vi "Calibration Axis.vi"() -> ()   [LabVIEW 2016]
doc: "This example builds a local coordinate system based on the information returned by an X-Y-Theta positioning system. The example finds the location of the template in the image and transforms the coordinates from the image coordinate system to the local system using the IMAQ Convert Pixel to Real World VI."
uses:
  <vilib>/vision/Calibration.llb/Error Statistics.ctl
  <vilib>/vision/NI_Vision_Development_Module.lvlib
panel:
  out "Calibration Axis Info":T1={"Origin Pixel"={"X"=0.0, "Y"=0.0}, "Angle Relative to Horizontal (deg)"=0.0, "X Axis Pixel"={"X"=0.0, "Y"=0.0}, "Axis Reference"=1} {"X Axis Pixel"."Y" format="%.2f"; "X Axis Pixel"."X" format="%.2f"; "Axis Reference" items=["Direct", "Indirect"]; "Angle Relative to Horizontal (deg)" format="%.2f"; "Origin Pixel"."Y" format="%.2f"; "Origin Pixel"."X" format="%.2f"}
  out "Error Statistics":T2
  out "Error Map":sgl[][](array[numeric]) format="%.2f"
  out "Board Mounting \nHole Location":T3 {"Calibration Axis (mm)"."Y" format="%#_2g"; "Calibration Axis (mm)"."X" format="%#_2g"}
  out "Calibration Axis":T4={"Origin Point (pixels)"={"X"=0.0, "Y"=0.0}, "Angle (degrees)"=0.0, "Axis Reference"=1} {"Axis Reference" items=["Direct", "Indirect"]; "Angle (degrees)" format="%.2f"; "Origin Point (pixels)"."Y" format="%.2f"; "Origin Point (pixels)"."X" format="%.2f"}
  out "Board Corner Template":T5(plugin-control)
  out "Mounting Hole Template":T5(plugin-control)
  out "Image":T5(plugin-control)
  # "Overview: Demonstrates how to use the Calibration functions to apply a simple calibration to an image, update the calibration axis as the part moves, and calculate the real world position of a feature compared with the pixel position of that same feature. \nRequirements: Vision Development Software.\nInstructions: Run the VI."
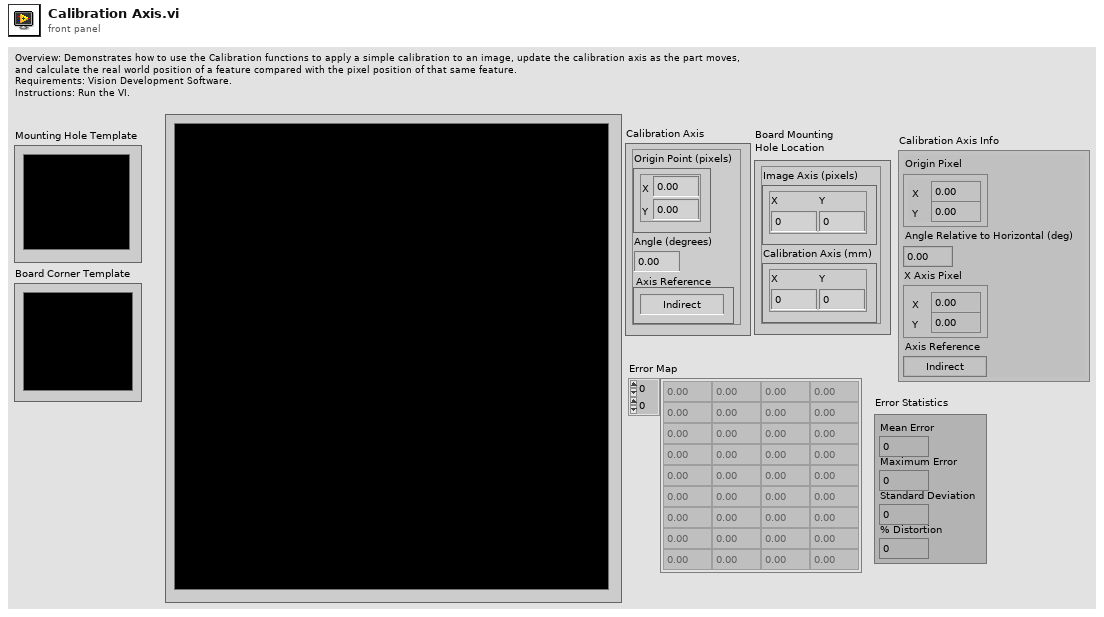
[diagram p1: front panel]
types:
  T1 = cluster{"Origin Pixel":cluster{"X":sgl, "Y":sgl}, "Angle Relative to Horizontal (deg)":sgl, "X Axis Pixel":cluster{"X":sgl, "Y":sgl}, "Axis Reference":u32}
  T2 = typedef "Error Statistics.ctl" = cluster{"Mean Error":dbl, "Maximum Error":dbl, "Standard Deviation":dbl, "% Distortion":dbl}
  T3 = cluster{"Image Axis (pixels)":cluster{"X":dbl, "Y":dbl}, "Calibration Axis (mm)":cluster{"X":dbl, "Y":dbl}}
  T4 = cluster{"Origin Point (pixels)":cluster{"X":sgl, "Y":sgl}, "Angle (degrees)":sgl, "Axis Reference":u32}
  T5 = typedef "IMAQ Image.ctl" = refnum<image>
  T6 = typedef "Image Type" = u32
  T7 = typedef "Simple Grid Descriptor" = cluster{"X Step":sgl, "Y Step":sgl, "Unit":T8}
  T8 = typedef "Image Unit" = enum32{"Undefined", "Angström", "Micrometer", "Millimeter", "Centimeter", "Meter", "Kilometer", "Microinch", "Inch", "Feet", "Nautical miles", "Standard miles", "Steps"}
  T9 = cluster{"Number of Matches Requested":i32, "Minimum Match Score":sgl, "Angle Ranges":cluster{"Start Angle":sgl, "End Angle":sgl}[]}
  T10 = cluster{"Position":cluster{"x":sgl, "y":sgl}, "Angle":sgl, "Scale":sgl, "Score":sgl, "Bounding Box":cluster{"x":sgl, "y":sgl}[]}[]
  T11 = cluster{"Position":cluster{"x":sgl, "y":sgl}, "Angle":sgl, "Scale":sgl, "Score":sgl, "Bounding Box":cluster{"x":sgl, "y":sgl}[]}
  T12 = cluster{"Position":cluster{"x":sgl, "y":sgl}, "Angle":sgl, "Axis Reference":u32}
  T13 = cluster{"Position":cluster{"x":sgl, "y":sgl}, "Real World Coordinates":cluster{"X":sgl, "Y":sgl}}
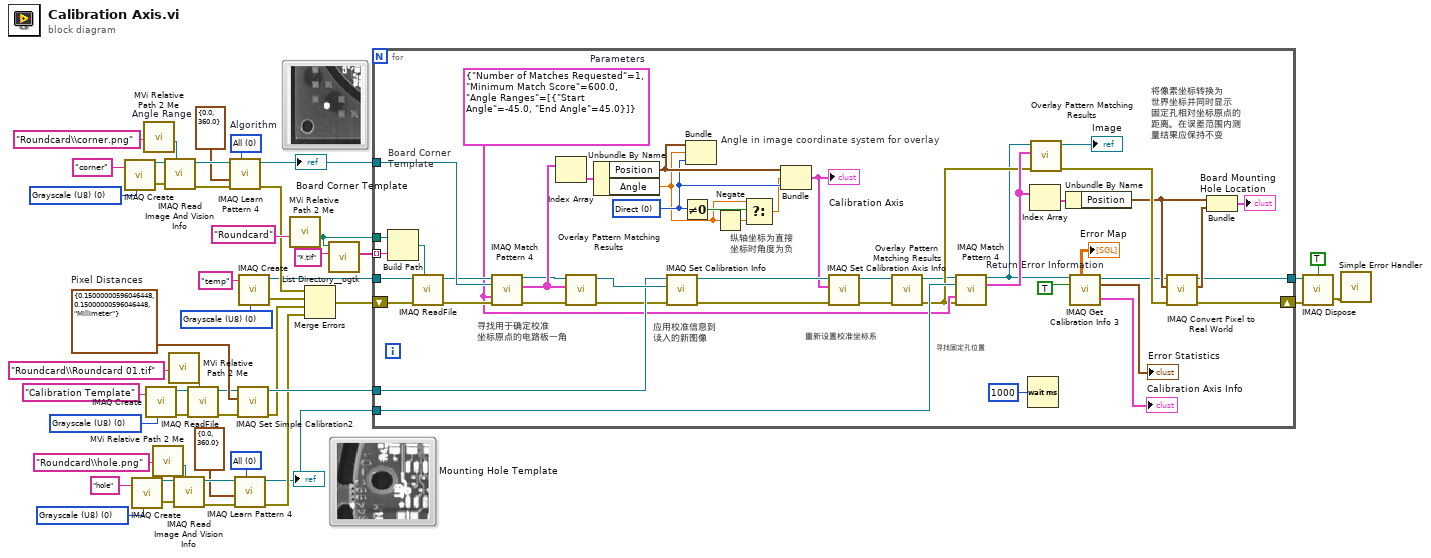
[diagram p0: block diagram]
diagram:
  w6 = 0 items=["All", "Low Discrepancy Sampling", "Grayscale Value Pyramid", "Gradients Pyramid"] ("Algorithm")
  w14 = T6 0 items=["Grayscale (U8)", "Grayscale (I16)", "Grayscale (SGL)", "Complex (CSG)", "RGB (U32)", "HSL (U32)", "RGB (U64)", "Grayscale (U16)"] ("Image Type")
  w24 = cluster{"Start Angle":sgl, "End Angle":sgl} {"Start Angle"=0.0, "End Angle"=360.0}  # Angle Range
  w7 = 0 items=["All", "Low Discrepancy Sampling", "Grayscale Value Pyramid", "Gradients Pyramid"]  # Algorithm
  w38 = T7 {"X Step"=0.15, "Y Step"=0.15, "Unit"=enum."Millimeter"}  # Pixel Distances
  w40 = T6 0 items=["Grayscale (U8)", "Grayscale (I16)", "Grayscale (SGL)", "Complex (CSG)", "RGB (U32)", "HSL (U32)", "RGB (U64)", "Grayscale (U16)"] ("Image Type")
  w43 = T6 0 items=["Grayscale (U8)", "Grayscale (I16)", "Grayscale (SGL)", "Complex (CSG)", "RGB (U32)", "HSL (U32)", "RGB (U64)", "Grayscale (U16)"] ("Image Type")
  w44 = T6 0 items=["Grayscale (U8)", "Grayscale (I16)", "Grayscale (SGL)", "Complex (CSG)", "RGB (U32)", "HSL (U32)", "RGB (U64)", "Grayscale (U16)"] ("Image Type")
  n1 = call "IMAQ Create"("Image Name"="corner" ("name or relative path"), "Image Type"=w43) -> ("Src"=w42:T5, "error out"=w41:errorcluster)  [unwired: 2 in, 1 out]
  n2 = call "IMAQ Create"("Image Name"="hole" ("name or relative path"), "Image Type"=w44) -> ("Src"=w47:T5, "error out"=w48:errorcluster)  [unwired: 2 in, 1 out]
  n3 = call "MVi Relative Path 2 Me.vi"("Relative Path"="Roundcard\\corner.png" ("name or relative path")) -> ("Appended Dir"=w20:path)  [unwired: 5 in, 1 out]
  n4 = call "IMAQ Create"("Image Name"="Calibration Template", "Image Type"=w40) -> ("Src"=w35:T5, "error out"=w32:errorcluster)  [unwired: 2 in, 1 out]
  n5 = call "MVi Relative Path 2 Me.vi"("Relative Path"="Roundcard\\hole.png" ("name or relative path")) -> ("Appended Dir"=w18:path)  [unwired: 5 in, 1 out]
  n6 = call "IMAQ Read Image And Vision Info"("File Path"=w20, "error in (no error)"=w41, "Image"=w42) -> ("error out"=w29:errorcluster, "Image Out"=w28:T5)  [unwired: 1 in, 6 out]
  n7 = call "MVi Relative Path 2 Me.vi"("Relative Path"="Roundcard\\Roundcard 01.tif" ("name or relative path")) -> ("Appended Dir"=w15:path)  [unwired: 5 in, 1 out]
  n8 = call "IMAQ Read Image And Vision Info"("File Path"=w18, "error in (no error)"=w48, "Image"=w47) -> ("error out"=w25:errorcluster, "Image Out"=w26:T5)  [unwired: 1 in, 6 out]
  n9 = call "IMAQ ReadFile"("File Path"=w15, "error in (no error)"=w32, "Image"=w35) -> ("error out"=w34:errorcluster, "Image Out"=w30:T5)  [unwired: 4 in, 3 out]
  n10 = call "IMAQ Learn Pattern 4"("Algorithm"=w7, "error in (no error)"=w29, "Angle Range"=w24, "Image"=w28) -> ("error out"=w12:errorcluster, "Template Image Out"=w27:T5)  [unwired: 5 in, 1 out]
  "Board Corner Template" <- w27
  n11 = call "IMAQ Learn Pattern 4"("Algorithm"=w6, "error in (no error)"=w25, "Angle Range"=cluster{"Start Angle":sgl, "End Angle":sgl} {"Start Angle"=0.0, "End Angle"=360.0}, "Image"=w26) -> ("error out"=w3:errorcluster, "Template Image Out"=w1:T5)  [unwired: 5 in, 1 out]
  "Mounting Hole Template" <- w1
  n12 = call "IMAQ Set Simple Calibration2"("error in (no error)"=w34, "Pixel Distances"=w38, "Image"=w30) -> ("error out"=w4:errorcluster, "Calibration Template Image"=w37:T5)  [unwired: 7 out]
  n13 = call "IMAQ Create"("Image Name"="temp", "Image Type"=w14) -> ("Src"=w11:T5, "error out"=w5:errorcluster)  [unwired: 2 in, 1 out]
  n14 = call "MVi Relative Path 2 Me.vi"("Relative Path"="Roundcard" ("name or relative path")) -> ("Appended Dir"=w10:path)  [unwired: 5 in, 1 out]
  n15 = Merge Errors(w12, w5, w4, w3) -> (w31:errorcluster)
  n16 = call "List Directory__ogtk.vi"("pattern"="*.tif", "directory path"=w10) -> ("file names"=w22:string[])  [unwired: 2 in, 3 out]
  n17 = for {
    tunnel: [w62] -> w46
    tunnel: w37 -> [w87]
    shift-right: [w61] -> w45
    shift-left: w31 -> [w76]
    tunnel: w27 -> [w78]
    tunnel: w22 -> [w72] mode=indexing
    tunnel: w11 -> [w74]
    tunnel: w10 -> [w71]
    tunnel: w1 -> [w63]
    w54 = T9 {"Number of Matches Requested"=1, "Minimum Match Score"=600.0, "Angle Ranges"=[{"Start Angle"=-45.0, "End Angle"=45.0}]}  # Parameters
    w55 = TRUE  # Return Error Information
    w69 = u32 0 items=["Direct", "Indirect"] ("Axis Reference")
    # "Board Corner\nTemplate"
    # "将像素坐标转换为\n世界坐标并同时显示\n固定孔相对坐标原点的\n距离。在误差范围内测\n量结果应保持不变"
    # "寻找固定孔位置"
    # "重新设置校准坐标系"
    # "应用校准信息到\n读入的新图像"
    # "寻找用于确定校准\n坐标原点的电路板一角"
    # "纵轴坐标为直接\n坐标时角度为负"
    # "Angle in image coordinate system for overlay"
    n18 = Build Path(base path=w71, name or relative path=w72) -> (appended path=w70:path)
    n19 = call "IMAQ ReadFile"("File Path"=w70, "error in (no error)"=w76, "Image"=w74) -> ("error out"=w75:errorcluster, "Image Out"=w73:T5)  [unwired: 4 in, 3 out]
    n20 = call "IMAQ Match Pattern 4"("Image"=w73, "Template Image"=w78, "Parameters"=w54, "error in (no error)"=w75) -> ("Image (duplicate)"=w64:T5, "Matches (pixel)"=w89:T10, "error out"=w84:errorcluster)  [unwired: 7 in, 2 out]
    n21 = Index Array(array=w89) -> (element=w90:T11)  [unwired: 1 in]
    n22 = call "Overlay Pattern Matching Results.vi"("error in"=w84, "Matches"=w89, "Image"=w64) -> ("error out"=w83:errorcluster, "Image Out"=w88:T5)  [unwired: 7 in]
    n23 = Unbundle By Name(w90) -> ("Position"=w86:cluster{"x":sgl, "y":sgl}, "Angle"=w67:sgl)
    n24 = call "IMAQ Set Calibration Info"("error in (no error)"=w83, "Image Dst"=w88, "Image Src"=w87) -> ("error out"=w92:errorcluster, "Calibrated Image"=w91:T5)  [unwired: 1 in, 6 out]
    n25 = Not Equal To 0?(x=w69) -> (x != 0?=w68:bool)
    n26 = Bundle("Position"=w86, "Angle"=w67, "Axis Reference"=w69) -> ()  [unwired: 2 out]
    n27 = Negate(x=w67) -> (-x=w66:sgl)
    n28 = Select(t=w67, s=w68, f=w66) -> (s? t:f=w65:sgl)
    n29 = Bundle("Position"=w86, "Angle"=w65, "Axis Reference"=w69) -> (w85:T12)  [unwired: 1 out]
    "Calibration Axis" <- w85
    n30 = call "IMAQ Set Calibration Axis Info"("error in (no error)"=w92, "Calibration Axis Info"=w85, "Calibration Template Image In"=w91) -> ("error out"=w53:errorcluster, "Calibration Template Image Out"=w52:T5)  [unwired: 7 out]
    n31 = call "Overlay Pattern Matching Results.vi"("error in"=w53, "Image"=w52) -> ("error out"=w51:errorcluster, "Image Out"=w50:T5)  [unwired: 3 in, 5 out]
    n32 = call "IMAQ Match Pattern 4"("Image"=w50, "Template Image"=w63, "Parameters"=w54, "error in (no error)"=w51) -> ("Image (duplicate)"=w49:T5, "Matches (pixel)"=w77:T10)  [unwired: 7 in, 3 out]
    n33 = Wait (ms)(milliseconds to wait=u32 1000) -> ()  [unwired: 1 out]
    n34 = Index Array(array=w77) -> (element=w94:T11)  [unwired: 1 in]
    n35 = call "Overlay Pattern Matching Results.vi"("error in"=w51, "Matches"=w77, "Image"=w49) -> ("error out"=w82:errorcluster, "Image Out"=→"Image":T5)  [unwired: 7 in]
    n36 = Unbundle By Name(w94) -> ("Position"=w81:cluster{"x":sgl, "y":sgl})
    n37 = call "IMAQ Get Calibration Info 3"("Calibration Template Image"=w49, "Return Error Information (False)"=w55) -> ("Error Map"=→"Error Map":sgl[][], "Calibration Template Image (duplicate)"=w57:T5, "Error Statistics"=→"Error Statistics":T2, "Calibration Axis Info"=→"Calibration Axis Info":T1)  [unwired: 5 in, 5 out]
    n38 = call "IMAQ Convert Pixel to Real World"("error in (no error)"=w82, "Pixel Coordinates"=w81, "Calibrated Image"=w57) -> ("error out"=w61:errorcluster, "Real World Coordinates"=w80:cluster{"X":sgl, "Y":sgl}, "Calibrated Image (duplicate)"=w62:T5)  [unwired: 1 in, 5 out]
    n39 = Bundle("Position"=w81, "Real World Coordinates"=w80) -> (→"Board Mounting \nHole Location":T13)  [unwired: 1 in]
  }
  n40 = call "IMAQ Dispose"("All Images? (No)"=TRUE, "Image"=w46, "error in (no error)"=w45) -> ("error out"=w8:errorcluster)  [unwired: 3 out]
  n41 = call <vilib>:"Simple Error Handler.vi"("error in (no error)"=w8) -> ()  [unwired: 1 in, 8 out]
